vi "Test 1.vi"() -> ()   [LabVIEW 2014, in "Generic Digital Multi Meter.lvlib" / "Tektronix DMM4020.lvlib" / "Tektronix DMM4020.lvclass"]
uses:
  Tektronix DMM4020.lvclass
  Controls/Numeric Indicator.ctl
  Abstract Sensor/Abstract Sensor.lvclass
  <vilib>/ActorFramework/Message Enqueuer/Message Enqueuer.lvclass/Message Enqueuer.ctl
  <vilib>/ActorFramework/Message Enqueuer/Enqueue.vi
  <vilib>/ActorFramework/Message Priority Queue/Priority Enqueue.vi
  <vilib>/ActorFramework/Stop Msg/Stop Msg.lvclass
  Abstract Sensor Messages/Measure Msg/Measure Msg.lvclass
  SetUp VIs/SetUp VIs.lvlib
  <vilib>/ActorFramework/Actor/Actor.lvclass
  <instrlib>/Tektronix DMM4020/Tektronix DMM4020.lvlib
  Display Panel/Display Panel V3/Display Panel V3.lvclass
panel:
  in  "Waveform Chart":dynamicdata(graph)
  out "Array":T1[](array[typedef])
  in  "Measure":bool
  in  "Stop Button":bool
  out "Manufacturer":string
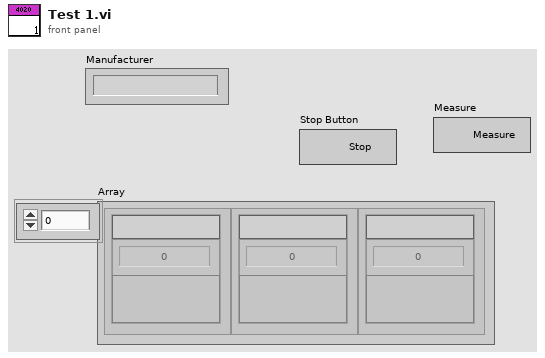
[diagram p1: front panel]
types:
  T1 = typedef "Numeric Indicator.ctl" = cluster{"Value":dbl, "Name":string, "Graph Button":bool}
  T2 = typedef "Instrument ID Object.ctl" = cluster{"Manufacturer":string, "Model":string, "Serial":string, "Address":string, "Select?":bool}
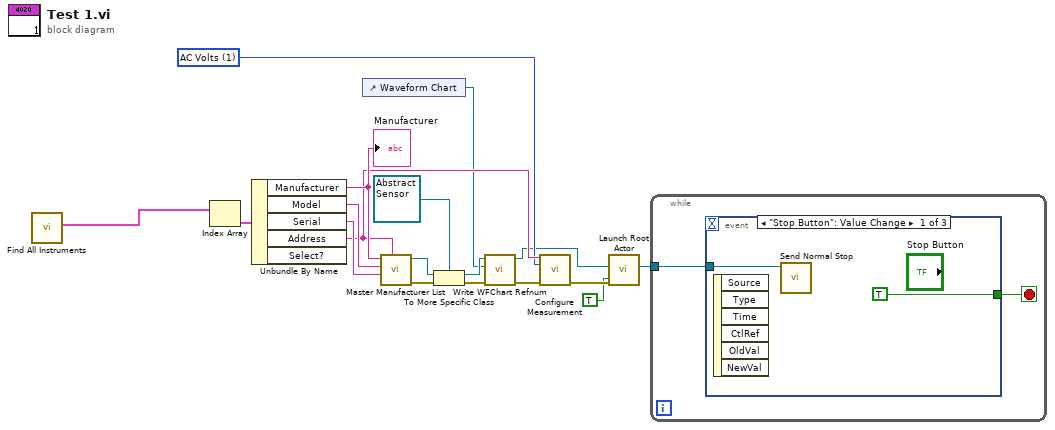
[diagram p0: block diagram]
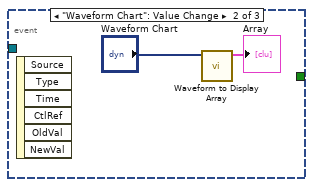
[diagram p2: hidden frame]
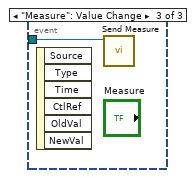
[diagram p3: hidden frame]
diagram:
  w11 = u16 1 items=["DC Volts", "AC Volts", "DC Current", "AC Current", "2-Wire Resistance", "4-Wire Resistance", "Frequency", "AC and DC rms Current", "AC and DC rms Volts", "Continuity", "Diode"] ("Measurement Function (0: DC Volts)")
  n1 = call "Find All Instruments.vi"() -> ("List of Instruments Out"=w18:T2[])  [unwired: 9 in, 2 out]
  n2 = Index Array(array=w18) -> (element=w17:T2)  [unwired: 1 in]
  n3 = Unbundle By Name(w17) -> ("Manufacturer"=w16:string, "Model"=w15:string, "Serial"=w14:string, "Address"=w12:string)  [unwired: 1 out]
  "Manufacturer" <- w16
  n4 = control-ref of="Waveform Chart"() -> (w1:refnum<vi>)
  n5 = call "Master Manufacturer List.vi"("VISA resource name"=w12, "Serial"=w14, "Model"=w15, "Manufacturer"=w16) -> ("error out"=w3:errorcluster, "Generic Instrument out"=w7:refnum<class "Generic Instrument.lvclass">)  [unwired: 6 in]
  n6 = To More Specific Class(target class=refnum<class "Abstract Sensor.lvclass"> refnum ("Abstract Sensor.lvlib:Abstract Sensor.lvclass"), reference=w7, error in=w3) -> (specific class reference=w5:refnum<class "Abstract Sensor.lvclass">, error out=w2:errorcluster)
  n7 = call-dynamic "Write WFChart Refnum.vi"("error in (no error)"=w2, "WFChart Refnum"=w1, "Abstract Sensor in"=w5) -> ("error out"=w4:errorcluster, "Abstract Sensor out"=w8:refnum<class "Abstract Sensor.lvclass">)  [unwired: 7 in]
  n8 = call <instrlib>:"Configure Measurement.vi"("VISA resource name"=w12, "Measurement Function (0: DC Volts)"=w11, "error in (no error)"=w4) -> ("error out"=w10:errorcluster)  [unwired: 11 in, 1 out]
  n9 = call <vilib>:"Launch Root Actor.vi"("Open Actor Core front panel? (F)"=TRUE, "error in (no error)"=w10, "Actor"=w8) -> ("Actor's Enqueuer"=w13:refnum<class "Message Enqueuer.lvclass">)  [unwired: 7 in, 1 out]
  n10 = while {
    tunnel: w13 -> [w20]
    stop <- w19 stop-if-true
    n11 = event shown="[0] \"Stop Button\": Value Change" {
      selector: _ -> [_ _ _]
      dyn-events: _ -> [_ _ _]
      timeout: _ -> [_ _ _]
      tunnel: w20 -> [w22 _ w25]
      tunnel: [TRUE _ _] -> w19
      event "Stop Button": Value Change {
        n12 = event-data() -> ()  [unwired: 1 in, 6 out]
        n13 = call <vilib>:"Send Normal Stop.vi"("Message Enqueuer"=w22) -> ()  [unwired: 10 in, 1 out]
      }
      event "Waveform Chart": Value Change {
        n14 = event-data() -> ()  [unwired: 1 in, 6 out]
        n15 = call "Waveform to Display Array.vi"("Waveform Chart"="Waveform Chart") -> ("Array"=→"Array":T1[])  [unwired: 9 in, 1 out]
      }
      event "Measure": Value Change {
        n16 = event-data() -> ()  [unwired: 1 in, 6 out]
        n17 = call "Send Measure.vi"("Message Enqueuer"=w25) -> ()  [unwired: 9 in, 2 out]
      }
    }
  }
